vi "New F-String Formatter.vi"(6 "include namespaces? (F)":bool, 8 "length (-1: Full)":i32=-1, 9 "# of callers (-1: All)":i32=-1, 10 "delimiter (\" > \")":string=" > ", 11 "format string (\"%T | %L | %M\")":string="%^<%Y-%m-%dT%H:%M:%S%3uZ>T | %-8L | %M") -> (3 "new f-string formatter":refnum<class "Format String.lvclass">)   [LabVIEW 2018, in "GLog.lvlib" / "Format String.lvclass"]
uses:
  Format String.lvclass
  Format String.lvclass/Format String.ctl
panel:
  # "Connector Pane"
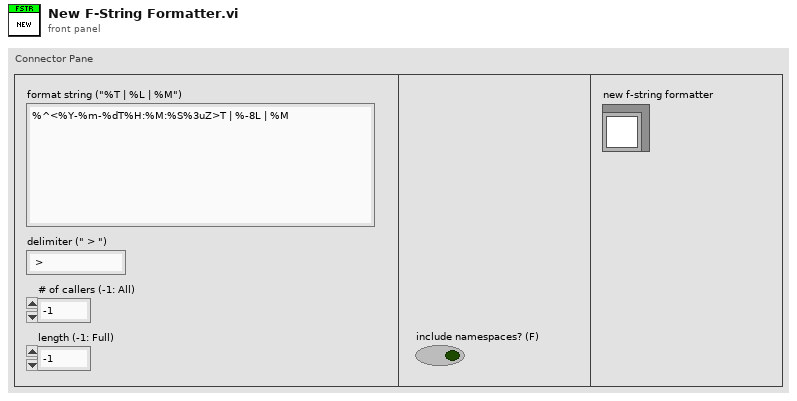
[diagram p1: front panel]
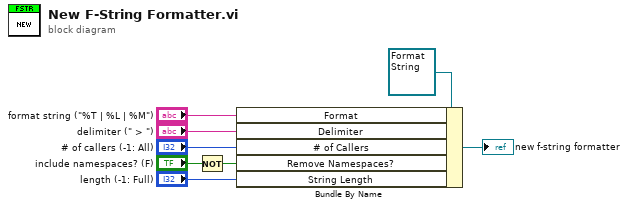
[diagram p0: block diagram]
diagram:
  n1 = Not(x="include namespaces? (F)") -> (.not. x?=w1:bool)
  n2 = Bundle By Name(cluster=refnum<class "Format String.lvclass"> refnum ("new f-string formatter"), "Format"="format string (\"%T | %L | %M\")", "Delimiter"="delimiter (\" > \")", "# of Callers"="# of callers (-1: All)", "Remove Namespaces?"=w1, "String Length"="length (-1: Full)") -> (→"new f-string formatter":refnum<class "Format String.lvclass">)
